vi "TCP Command Received.vi"(8 "error in (no error)":errorcluster, 9 "Message":string, 10 "GUID":string, 11 "tWorkerController in":refnum<class "tWorkerController.lvclass">) -> (0 "error out":errorcluster, 3 "tWorkerController out":refnum<class "tWorkerController.lvclass">)   [LabVIEW 2013, in "tWorkerController.lvlib" / "tWorkerController.lvclass"]
uses:
  tWorkerController.lvclass
  <vilib>/ActorFramework/Actor/Actor.lvclass/Actor.ctl
  LVAutomationListener/msgs/Log Event Msg/Log Event Msg.lvclass/Log Event Msg.ctl
  <vilib>/ActorFramework/Message Enqueuer/Message Enqueuer.lvclass/Message Enqueuer.ctl
  <vilib>/ActorFramework/Message Enqueuer/Enqueue.vi
  <vilib>/ActorFramework/Message Priority Queue/Priority Enqueue.vi
  LVAutomationListener/msgs/Log Event Msg/Log Event Msg.lvclass
  <vilib>/ActorFramework/Actor/Actor.lvclass
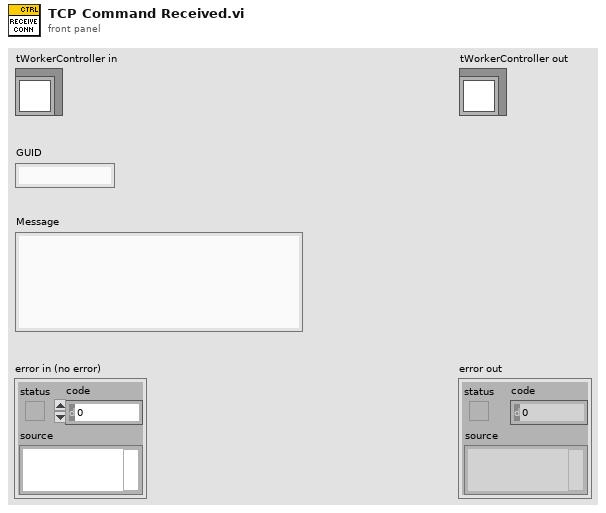
[diagram p1: front panel]
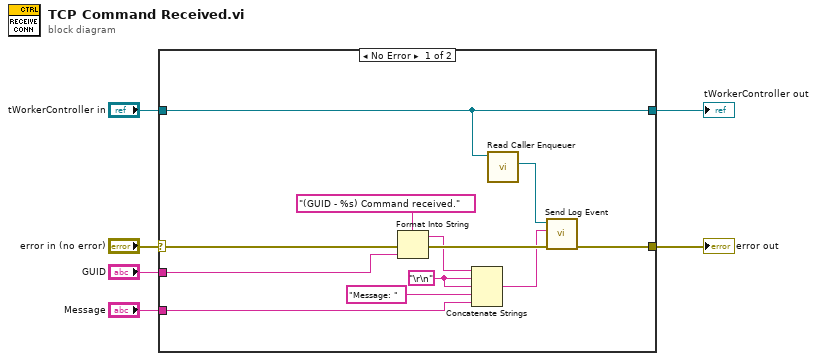
[diagram p0: block diagram]
diagram:
  n1 = case shown="No Error" "error in (no error)" {
    selector: "error in (no error)" -> [w15 w20]
    tunnel: [w17 w20] -> w4
    tunnel: [w18 w19] -> w5
    tunnel: "tWorkerController in" -> [w18 w19]
    tunnel: "GUID" -> [w16 _]
    tunnel: "Message" -> [w14 _]
    frame No Error {
      w7 = "\r\n"
      n2 = Format Into String(format string="(GUID - %s) Command received.", error in=w15, w16) -> (resulting string=w10:string, error out=w12:errorcluster)  [unwired: 1 in]
      n3 = Concatenate Strings(w10, w7, w7, "Message: " ("string"), w14) -> (w9:string)
      n4 = call <vilib>:"Read Caller Enqueuer.vi"("Actor"=w18) -> ("Caller Enqueuer"=w11:refnum<class "Message Enqueuer.lvclass">)  [unwired: 10 in]
      n5 = call "Send Log Event.vi"("error in (no error)"=w12, "Event Text"=w9, "Message Enqueuer"=w11) -> ("error out"=w17:errorcluster)  [unwired: 7 in, 1 out]
    }
    frame Error {
    }
  }
  "error out" <- w4
  "tWorkerController out" <- w5
